vi "Example5.vi"() -> ()   [LabVIEW 2019]
panel:
  out "Triggered":bool
  in  "Threshold":dbl
  in  "Slide":dbl(slide) scale=0.0..10.0
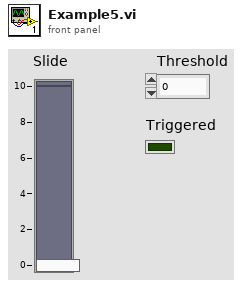
[diagram p1: front panel]
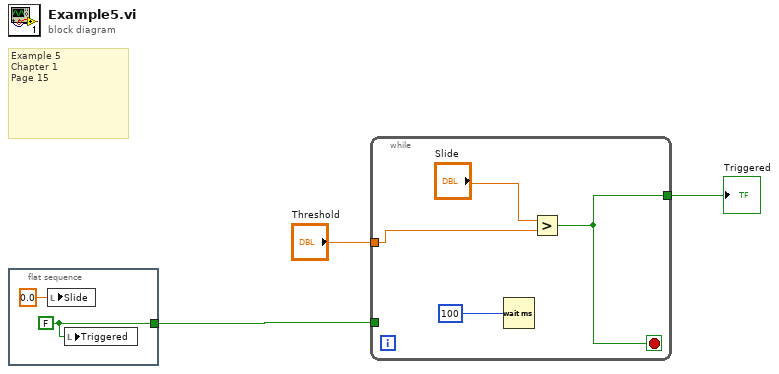
[diagram p0: block diagram]
diagram:
  # "Example 5\nChapter 1\nPage 15"
  n1 = flat-sequence {
    tunnel: [w4] -> w3
    frame #0 {
      w4 = FALSE ("Triggered")
      n2 = local write "Slide"(0.0 ("Slide")) -> ()
      n3 = local write "Triggered"(w4) -> ()
    }
  }
  n4 = while {
    tunnel: w3 -> [_]
    tunnel: "Threshold" -> [w7]
    tunnel: [w9] -> w1
    stop <- w9 stop-if-true
    n5 = Wait (ms)(milliseconds to wait=u32 100) -> ()  [unwired: 1 out]
    n6 = Greater?(x="Slide", y=w7) -> (0:w9:bool)
  }
  "Triggered" <- w1
